vi "blue screan logic.vi"(0 "DI":bool[](array[boolean]), 5 "DO":bool[](array[boolean]), 7 "AI":dbl[](array[numeric]), 9 "AO":dbl[](array[numeric]), 11 "Setting":T1) -> (4 "blue screan PMG":T2={"AI1"={"Numeric"=42.780748663101605, "Numeric"=31.016042780748666, "Numeric"=60.96256684491979}, "AI_0"={"Numeric"=57.25190839694657, "Numeric"=41.711229946524064, "Numeric"=72.19251336898397}, "AI_2"={"Numeric"=57.25190839694657, "Numeric"=35.82887700534759, "Numeric"=75.93582887700535}, "AI3"={"Numeric"=57.25190839694657, "Numeric"=41.711229946524064, "Numeric"=78.6096256684492}, "M24"=FALSE, "M24 pipe 1"=FALSE, "M24 pipe 2"=FALSE, "M24 pipe 3"=FALSE, "W 18.2"=FALSE, "W 18.2 pipe 2"=FALSE, "W 18.2 pipe 1"=FALSE, "W 18.2 tank"=FALSE, "M12"=FALSE, "M12 pipe 3"=FALSE, "M12 pipe 1"=FALSE, "M12 pipe 2"=FALSE, "M21"=FALSE, "M21 pipe 1"=FALSE, "M21 pipe 2"=FALSE, "M21 pipe 24"=FALSE, "M21 pipe 3"=FALSE, "W18.1"=FALSE, "W18.1 pipe 1"=FALSE, "W18.1 pipe 2"=FALSE, "W18.1 tank"=FALSE, "AO"=0.0} {"AI3" scale=0.0..100.0; "AI1" scale=0.0..100.0 scale format="%#.1f"; "AI_2" scale=0.0..100.0; "AI_0" scale=0.0..100.0})   [LabVIEW 2019, in "GUI PumpMotorGroup.lvclass"]
uses:
  GUI PumpMotorGroup.lvclass
  FPGA/TypeDef/blue screan PMG.ctl
  TypeDef/GUI Setting PMG.ctl
panel:
  # "НС Охлаждения и отчистки (М24)"
  # "НС Подачи масла (М21)"
  # "НС Перекачки масла (М12)"
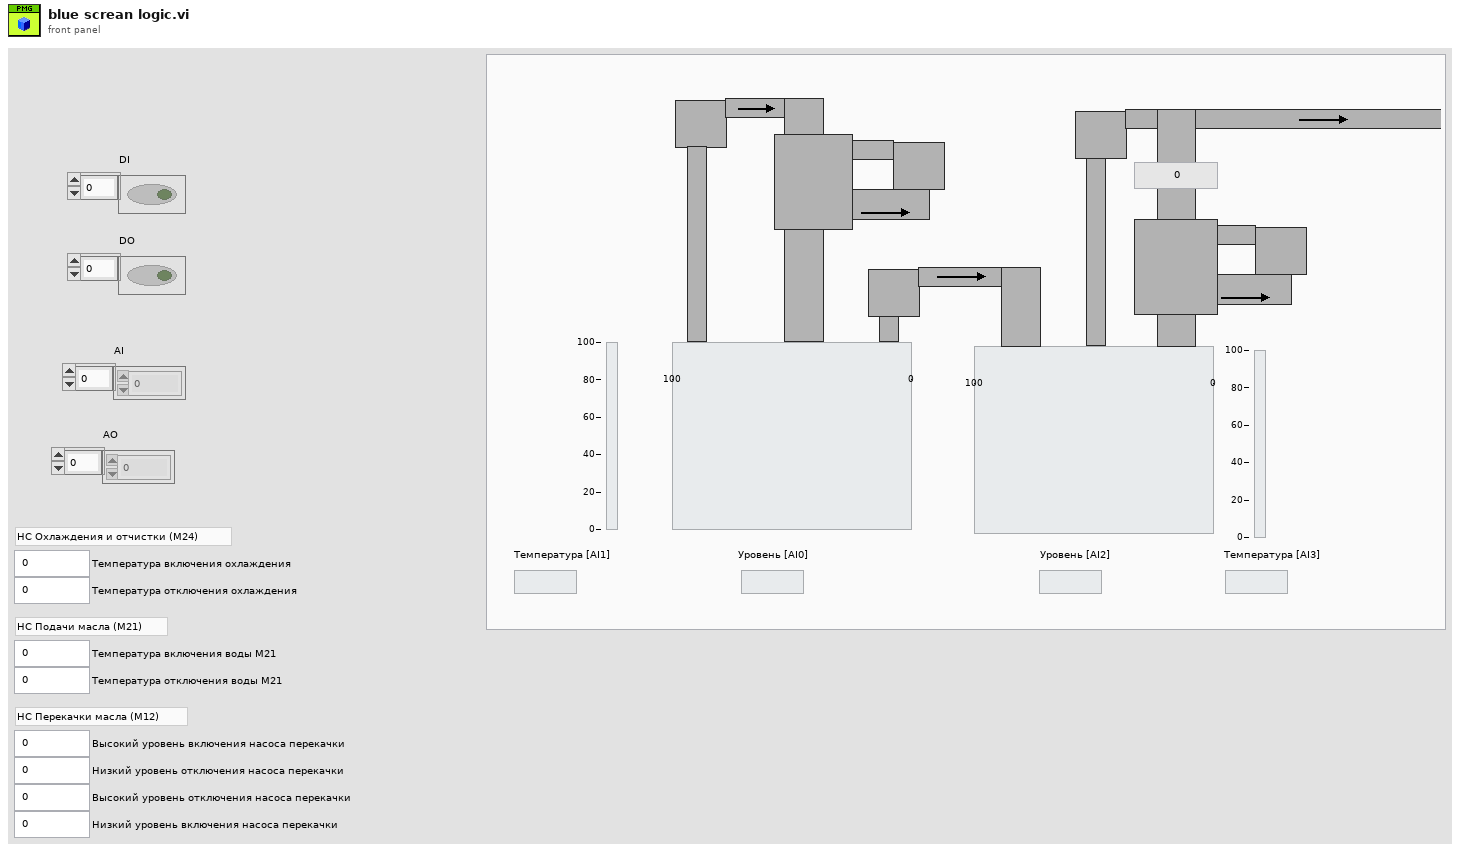
[diagram p1: front panel]
types:
  T1 = typedef "GUI Setting PMG.ctl" = cluster{"Temp Turn ON M24":dbl, "Temp Turn OFF M24":dbl, "Temp Open Water M21":dbl, "Temp Close Water M21":dbl, "H_51_on (cool)":dbl, "L_51_off (cool)":dbl, "H_52_off (oil)":dbl, "L_52_on (oil)":dbl}
  T2 = typedef "blue screan PMG.ctl" = cluster{"AI1":cluster{"Numeric":dbl, "Numeric":dbl, "Numeric":dbl}, "AI_0":cluster{"Numeric":dbl, "Numeric":dbl, "Numeric":dbl}, "AI_2":cluster{"Numeric":dbl, "Numeric":dbl, "Numeric":dbl}, "AI3":cluster{"Numeric":dbl, "Numeric":dbl, "Numeric":dbl}, "M24":bool, "M24 pipe 1":bool, "M24 pipe 2":bool, "M24 pipe 3":bool, "W 18.2":bool, "W 18.2 pipe 2":bool, "W 18.2 pipe 1":bool, "W 18.2 tank":bool, "M12":bool, "M12 pipe 3":bool, "M12 pipe 1":bool, "M12 pipe 2":bool, "M21":bool, "M21 pipe 1":bool, "M21 pipe 2":bool, "M21 pipe 24":bool, "M21 pipe 3":bool, "W18.1":bool, "W18.1 pipe 1":bool, "W18.1 pipe 2":bool, "W18.1 tank":bool, "AO":dbl}
  T3 = cluster{"DOs":dbl, "L_51_off (cool)":dbl, "H_51_on (cool)":dbl}
  T4 = cluster{"DOs":dbl, "Temp Turn OFF M24":dbl, "Temp Turn ON M24":dbl}
  T5 = cluster{"DOs":dbl, "L_52_on (oil)":dbl, "H_52_off (oil)":dbl}
  T6 = cluster{"DOs":dbl, "Temp Close Water M21":dbl, "Temp Open Water M21":dbl}
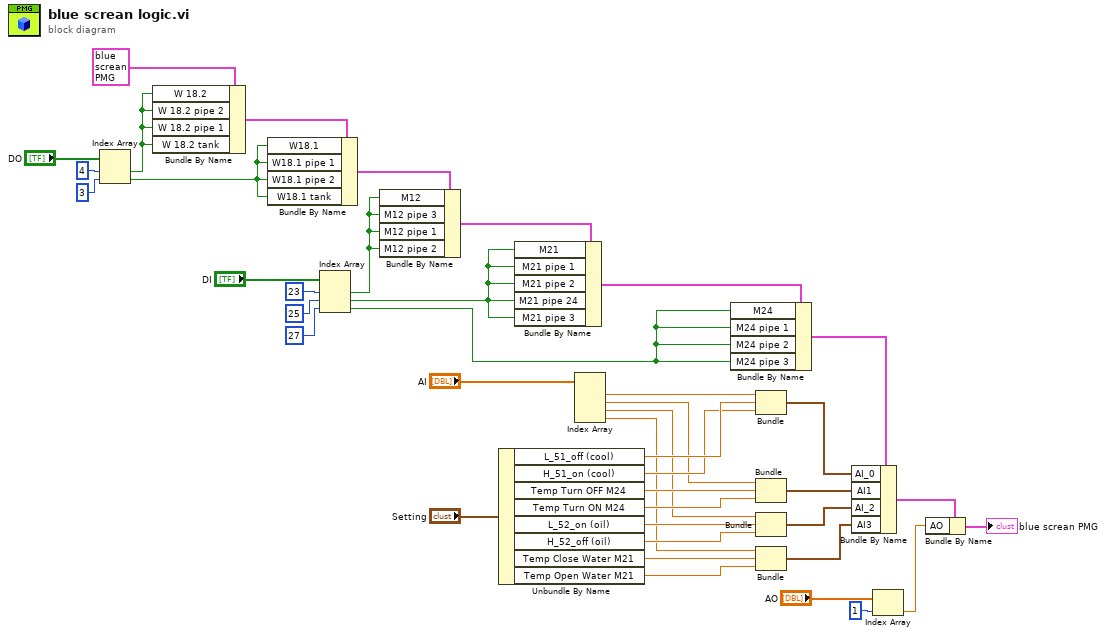
[diagram p0: block diagram]
diagram:
  n1 = Index Array(array="DO", index #1=4 ("index"), index #2=3 ("index")) -> (element #1=w39:bool, element #2=w36:bool)
  n2 = Bundle By Name(cluster=T2 {"AI1"={"Numeric"=42.780748663101605, "Numeric"=31.016042780748666, "Numeric"=60.96256684491979}, "AI_0"={"Numeric"=57.25190839694657, "Numeric"=41.711229946524064, "Numeric"=72.19251336898397}, "AI_2"={"Numeric"=57.25190839694657, "Numeric"=35.82887700534759, "Numeric"=75.93582887700535}, "AI3"={"Numeric"=57.25190839694657, "Numeric"=41.711229946524064, "Numeric"=78.6096256684492}, "M24"=FALSE, "M24 pipe 1"=FALSE, "M24 pipe 2"=FALSE, "M24 pipe 3"=FALSE, "W 18.2"=FALSE, "W 18.2 pipe 2"=FALSE, "W 18.2 pipe 1"=FALSE, "W 18.2 tank"=FALSE, "M12"=FALSE, "M12 pipe 3"=FALSE, "M12 pipe 1"=FALSE, "M12 pipe 2"=FALSE, "M21"=FALSE, "M21 pipe 1"=FALSE, "M21 pipe 2"=FALSE, "M21 pipe 24"=FALSE, "M21 pipe 3"=FALSE, "W18.1"=FALSE, "W18.1 pipe 1"=FALSE, "W18.1 pipe 2"=FALSE, "W18.1 tank"=FALSE, "AO"=0.0} ("blue screan PMG"), "W 18.2"=w39, "W 18.2 pipe 2"=w39, "W 18.2 pipe 1"=w39, "W 18.2 tank"=w39) -> (w37:T2)
  n3 = Bundle By Name(cluster=w37, "W18.1"=w36, "W18.1 pipe 1"=w36, "W18.1 pipe 2"=w36, "W18.1 tank"=w36) -> (w32:T2)
  n4 = Index Array(array="DI", index #1=23 ("index"), index #2=25 ("index"), index #3=27 ("index")) -> (element #1=w33:bool, element #2=w29:bool, element #3=w26:bool)
  n5 = Bundle By Name(cluster=w32, "M12"=w33, "M12 pipe 3"=w33, "M12 pipe 1"=w33, "M12 pipe 2"=w33) -> (w31:T2)
  n6 = Unbundle By Name("Setting") -> ("L_51_off (cool)"=w18:dbl, "H_51_on (cool)"=w17:dbl, "Temp Turn OFF M24"=w12:dbl, "Temp Turn ON M24"=w11:dbl, "L_52_on (oil)"=w8:dbl, "H_52_off (oil)"=w7:dbl, "Temp Close Water M21"=w4:dbl, "Temp Open Water M21"=w3:dbl)
  n7 = Bundle By Name(cluster=w31, "M21"=w29, "M21 pipe 1"=w29, "M21 pipe 2"=w29, "M21 pipe 24"=w29, "M21 pipe 3"=w29) -> (w28:T2)
  n8 = Index Array(array="AI") -> (element #1=w20:dbl, element #2=w13:dbl, element #3=w9:dbl, element #4=w5:dbl)  [unwired: 4 in]
  n9 = Bundle By Name(cluster=w28, "M24"=w26, "M24 pipe 1"=w26, "M24 pipe 2"=w26, "M24 pipe 3"=w26) -> (w24:T2)
  n10 = Bundle("DOs"=w20, "L_51_off (cool)"=w18, "H_51_on (cool)"=w17) -> (w16:T3)  [unwired: 1 in]
  n11 = Bundle("DOs"=w13, "Temp Turn OFF M24"=w12, "Temp Turn ON M24"=w11) -> (w10:T4)  [unwired: 1 in]
  n12 = Bundle("DOs"=w9, "L_52_on (oil)"=w8, "H_52_off (oil)"=w7) -> (w6:T5)  [unwired: 1 in]
  n13 = Bundle("DOs"=w5, "Temp Close Water M21"=w4, "Temp Open Water M21"=w3) -> (w2:T6)  [unwired: 1 in]
  n14 = Bundle By Name(cluster=w24, "AI_0"=w16, "AI1"=w10, "AI_2"=w6, "AI3"=w2) -> (w15:T2)
  n15 = Index Array(array="AO", index=1) -> (element=w14:dbl)
  n16 = Bundle By Name(cluster=w15, "AO"=w14) -> (→"blue screan PMG":T2)
